vi "Istwert abholen Position finden.vi"(7 "automatisch":bool, 8 "error in (no error)":errorcluster caption="Fehler (Eingang, kein Fehler)", 9 "Position Index in":i32=-1, 11 "Gasindex":i32) -> (0 "error out":errorcluster caption="Fehler (Ausgang)", 1 "Position Index out":i32, 3 "Gasindex out":i32)   [LabVIEW 2020, in "Linearisierung v2.lvlib"]
uses:
  Linearisierung v2.lvlib
  Aktion Lin Daten aufarbeiten.ctl
  Allgemein/allgemeine Sub-VIs.lvlib
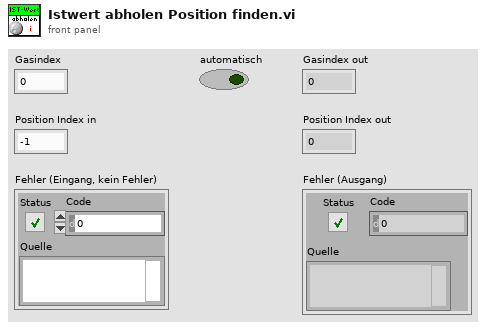
[diagram p1: front panel]
types:
  T1 = typedef "Linearisierung v2.lvlib/Aktion Lin Daten aufarbeiten.ctl" = enum16{"lesen", "Protkolldaten", "speichern", "laden", "EPA auswerten", "Tabelle schreiben", "Lin auswerten", "Tab init", "Stufentabelle", "EPA aktiviert", "Nachbehandlung laden", "Tabelle löschen", "Istwerte löschen", "Zeile löschen", "Zeile einfügen", "LIN aktiviert", "LIN/EPA aktiv laden", "EGAK Tab", "LIN übernehmen", "Tab init ohne Stufen"}
  T2 = typedef "Linearisierung v2.lvlib/Eingabetabelle.ctl" = string[][]
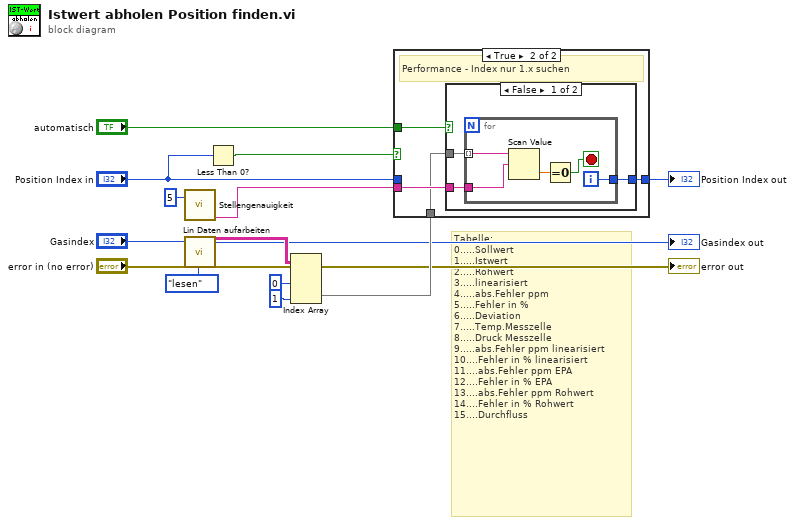
[diagram p0: block diagram]
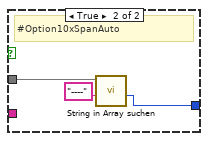
[diagram p3: hidden frame]
diagram:
  # "Tabelle:\n0.....Sollwert\n1.....Istwert\n2.....Rohwert\n3.....linearisiert\n4.....abs.Fehler ppm\n5.....Fehler in %\n6.....Deviation\n7.....Temp.Messzelle\n8.....Druck Messzelle\n9.....abs.Fehler ppm linearisiert\n10....Fehler in % linearisiert\n11....abs.Fehler ppm EPA\n12....Fehler in % EPA\n13....abs.Fehler ppm Rohwert\n14....Fehler in % Rohwert\n15....Durchfluss"
  n1 = call "Stellengenauigkeit.vi"("Genauigkeit (6)"=i16 5) -> ("Formatstring"=w11:string)  [unwired: 9 in, 1 out]
  n2 = call "Lin Daten aufarbeiten.vi"("Index (Seite)"="Gasindex", "error in (no error)"="error in (no error)", "Aktionen"=Aktion_Lin_Daten_aufarbeiten."lesen") -> ("Eingabetabelle"=w7:T2, "Index (Seite) out"=→"Gasindex out":i32, "error out"=→"error out":errorcluster)  [unwired: 14 in, 8 out]
  n3 = Less Than 0?(x="Position Index in") -> (x < 0?=w4:bool)
  n4 = Index Array(array=w7, index (col) #1=0 ("Deaktivierter Index (Spalte)"), index (col) #2=1 ("Deaktivierter Index (Spalte)")) -> (element #2=w9:string[])  [unwired: 2 in, 1 out]
  n5 = case shown="True" w4 {
    tunnel: w11 -> [_ w20]
    tunnel: "automatisch" -> [_ w19]
    tunnel: w9 -> [_ w18]
    tunnel: [w16 w17] -> w6
    tunnel: "Position Index in" -> [w16 _]
    frame False {
    }
    frame True {
      # "Performance - Index nur 1.x suchen"
      n6 = case shown="False" w19 {
        tunnel: w18 -> [w23 w30]
        tunnel: w20 -> [w22 _]
        tunnel: [w21 w29] -> w17
        frame False {
          n7 = for {
            tunnel: w23 -> [w27] mode=indexing
            tunnel: w22 -> [w28]
            tunnel: [w24] -> w21
            i -> [w24]
            stop <- w25 stop-if-true
            n8 = Scan Value(string=w27, format string=w28) -> (value=w26:dbl)  [unwired: 1 in, 1 out]
            n9 = Equal To 0?(x=w26) -> (x = 0?=w25:bool)
          }
        }
        frame True {
          # "#Option10xSpanAuto"
          n10 = call "String in Array suchen.vi"("Nach String/Zeichen suchen (-)"="----", "String-Array"=w30) -> ("Index"=w29:i32)  [unwired: 7 in, 2 out]
        }
      }
    }
  }
  "Position Index out" <- w6
